vi "Sprinkler.vi"() -> ()   [LabVIEW 2020]
uses:
  SubVIs/Machine States.ctl
  Controls/Control-Indicator References.ctl
panel:
  in  "Zone Setup Array":cluster{"Zone Selector":string, "Timing":dbl}[](array[cluster])
  out "Controller Status":string
  out "Zone Indicators":T1
  in  "Water Pressure Sensor (%)":u32(slide) scale=0.0..100.0
  in  "Rain Sensor":bool
  in  "Run Selector":bool
  in  "Setup":bool
  in  "Start":bool
  in  "stop":bool
  # "Controls"
  # "Simulation Controls"
  # "Rain"
  # "No Rain"
  # "Continuous"
  # "Single"
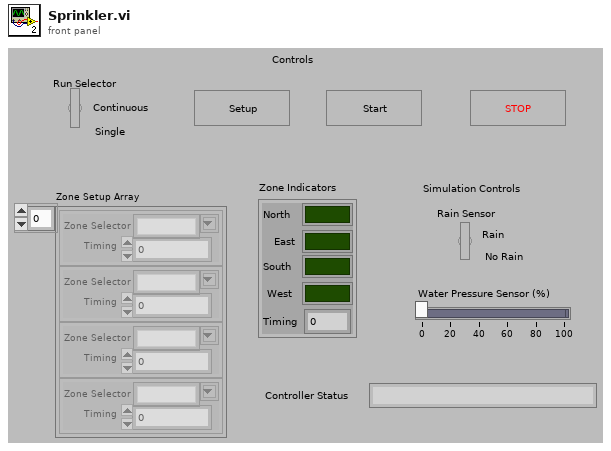
[diagram p1: front panel]
types:
  T1 = cluster{"North":bool, "East":bool, "South":bool, "West":bool, "Timing":u32}
  T2 = typedef "Control-Indicator References.ctl" = cluster{"Setup":refnum<vi>, "Start":refnum<vi>, "Controller Status":refnum<vi>, "Zone Setup Array":refnum<vi>, "Run Selector":refnum<vi>, "Rain Sensor":refnum<vi>, "Water Pressure Sensor (%)":refnum<vi>, "Zone Indicators":refnum<vi>}
  T3 = typedef "Machine States.ctl" = enum16{"Init", "Setup", "Start", "Stop", "Wait To Start", "Low Water Pressure", "Rain"}
  T4 = cluster{bool, bool, bool, bool, "Elapsed Time":dbl}
  T5 = enum8{"Enabled", "Disabled", "Disabled and Grayed Out"}
  T6 = typedef "Timer Controls.ctl" = enum16{"Reset", "Start", "Stop"}
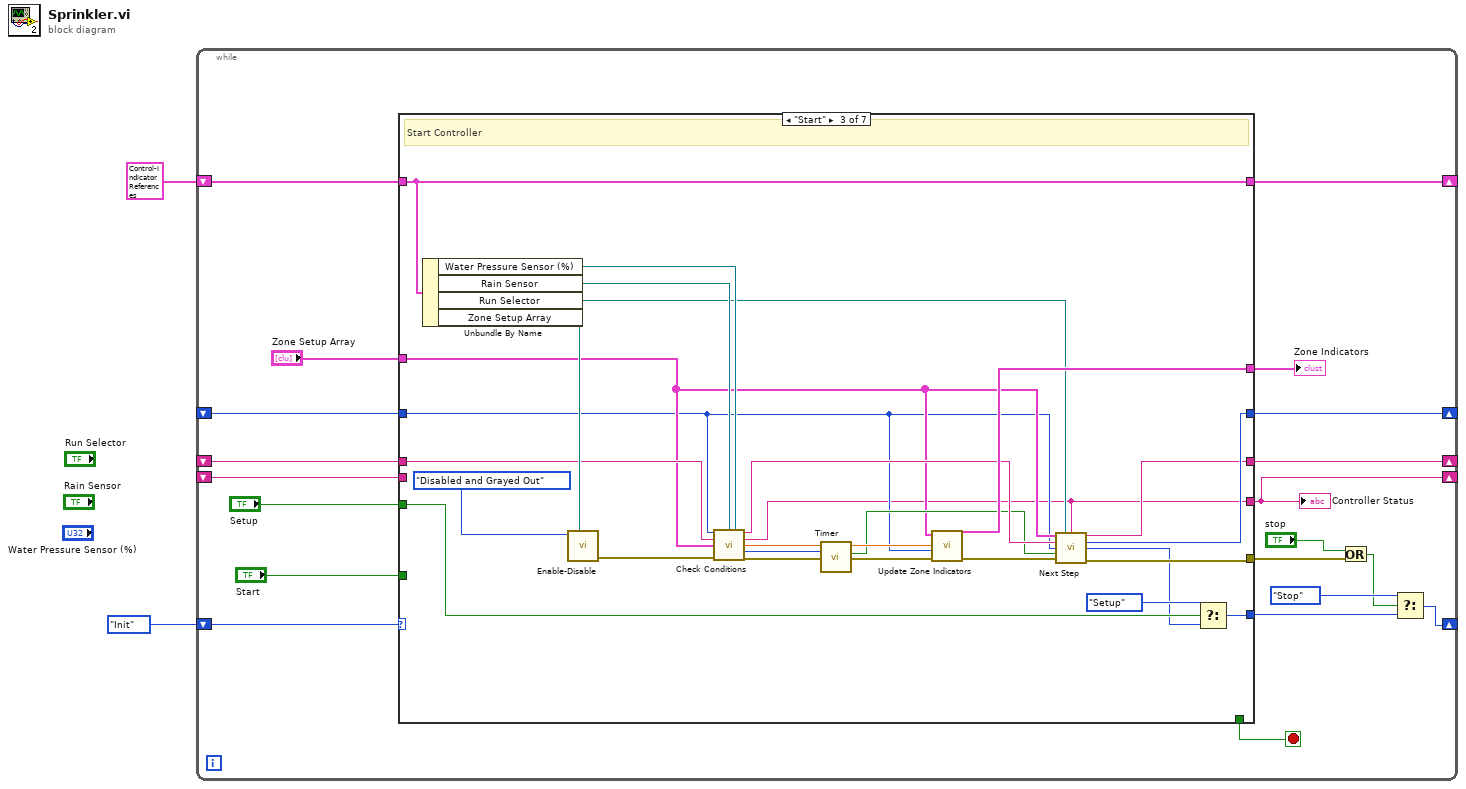
[diagram p0: block diagram]
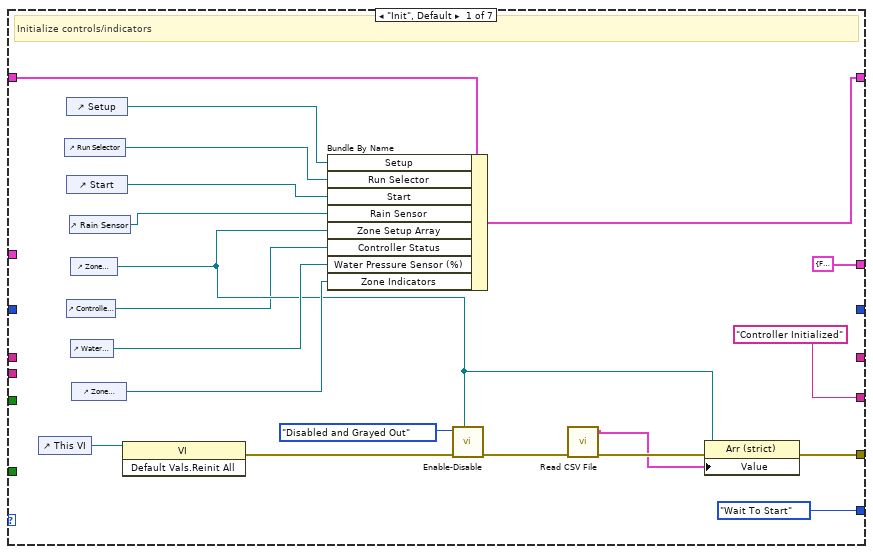
[diagram p2: hidden frame]
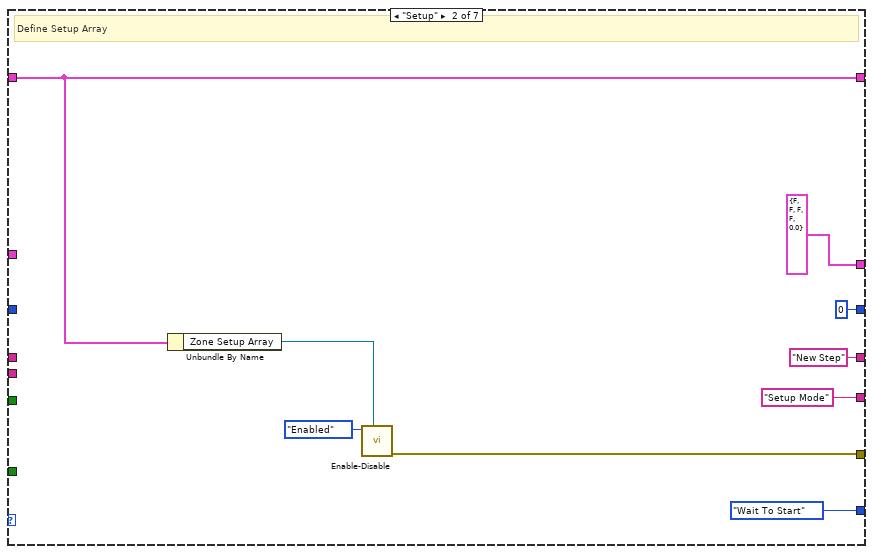
[diagram p3: hidden frame]
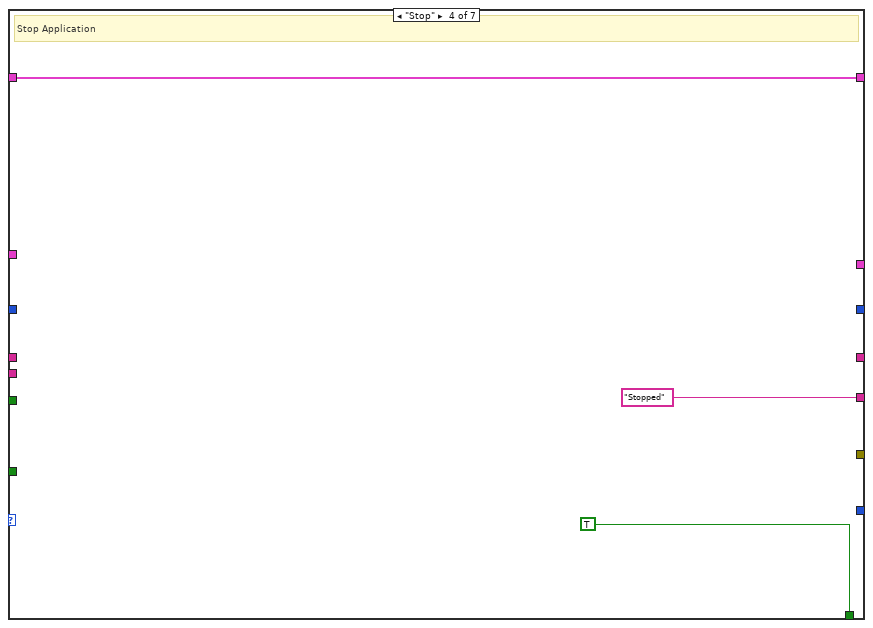
[diagram p4: hidden frame]
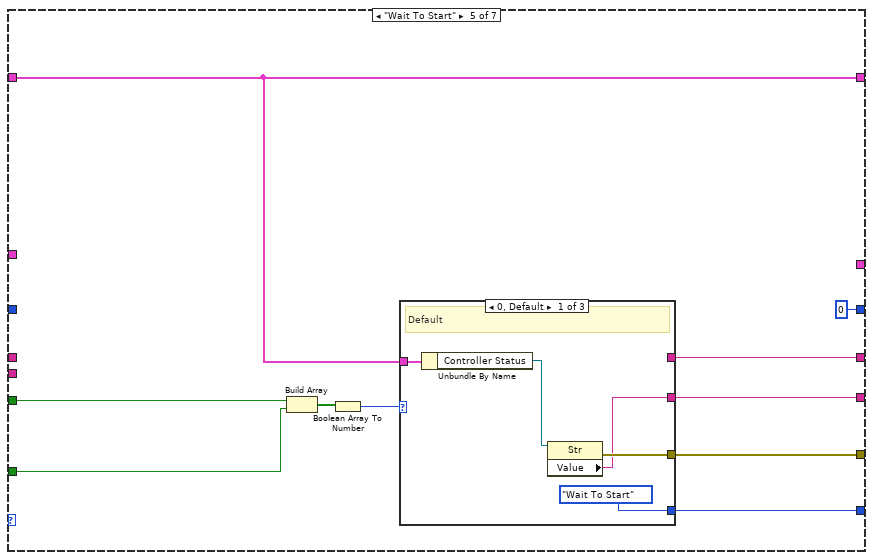
[diagram p5: hidden frame]
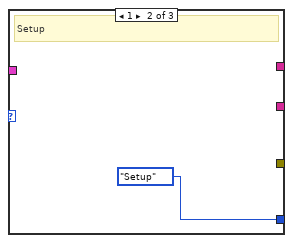
[diagram p6: hidden frame]
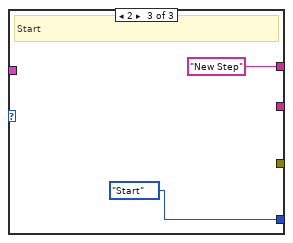
[diagram p7: hidden frame]
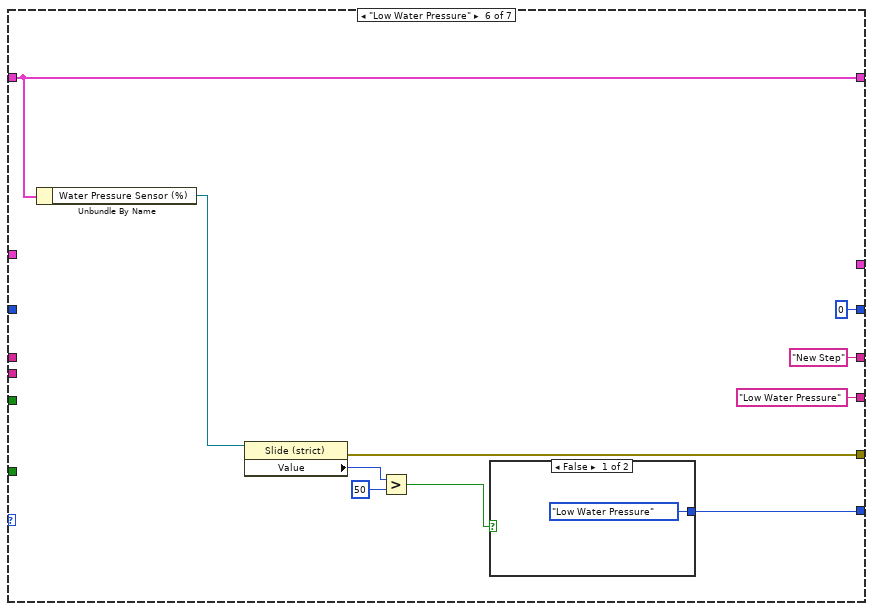
[diagram p8: hidden frame]
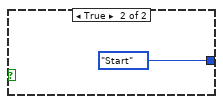
[diagram p9: hidden frame]
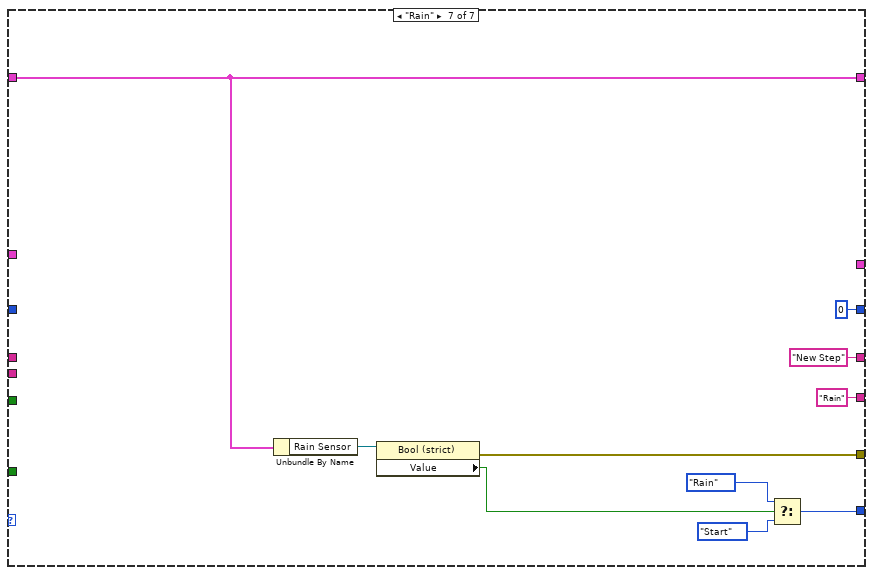
[diagram p10: hidden frame]
diagram:
  n1 = while {
    shift-right: [w18] -> _
    shift-left: Machine_States."Init" ("Enum") -> [w22]
    shift-right: [w11] -> _
    shift-left: T2 {"Setup"=refnum, "Start"=refnum, "Controller Status"=refnum, "Zone Setup Array"=refnum, "Run Selector"=refnum, "Rain Sensor"=refnum, "Water Pressure Sensor (%)"=refnum, "Zone Indicators"=refnum} -> [w21]
    shift-right: [w10] -> _
    shift-left: _ -> [w9]
    shift-right: [w7] -> _
    shift-left: _ -> [w6]
    shift-right: [w5] -> _
    shift-left: _ -> [w4]
    stop <- w17 stop-if-true
    n2 = case shown="\"Start\"" w22 {
      tunnel: w21 -> [w25 w49 w77 w78 w85 w100 w112]
      tunnel: ["Controller Initialized" ("Controller Status") "Setup Mode" ("Controller Status") w52 "Stopped" ("Controller Status") w83 "Low Water Pressure" ("Value") "Rain" ("Value")] -> w10
      tunnel: [w30 w51 w62 _ w84 w107 w116] -> w15
      tunnel: [Machine_States."Wait To Start" ("Enum") Machine_States."Wait To Start" ("f") w53 _ w86 w101 w117] -> w20
      tunnel: [_ _ _ TRUE _ _ _] -> w17
      tunnel: "Start" -> [_ _ _ _ w87 _ _]
      tunnel: "Setup" -> [_ _ w74 _ w90 _ _]
      tunnel: [w24 w49 w77 w78 w85 w100 w112] -> w11
      tunnel: w9 -> [_ _ _ _ _ _ _]
      tunnel: [_ "New Step" ("Step Status Out") w55 _ w81 "New Step" ("Step Status Out") "New Step" ("Step Status Out")] -> w7
      tunnel: "Zone Setup Array" -> [_ _ w57 _ _ _ _]
      tunnel: w6 -> [_ _ w67 _ _ _ _]
      tunnel: [_ 0 w60 _ 0 ("Step Out") 0 ("Step Out") 0 ("Step Out")] -> w5
      tunnel: w4 -> [_ _ w56 _ _ _ _]
      tunnel: [T4 {FALSE, FALSE, FALSE, FALSE, "Elapsed Time"=0.0} ("Zone Indicators") T4 {FALSE, FALSE, FALSE, FALSE, "Elapsed Time"=0.0} ("Zone Indicators") w64 _ _ _ _] -> w3
      frame "Init", Default {
        # "Initialize controls/indicators"
        n3 = control-ref of="This VI"() -> (w42:refnum<vi>)
        n4 = control-ref of="Run Selector"() -> (w40:refnum<vi>)
        n5 = control-ref of="Setup"() -> (w41:refnum<vi>)
        n6 = control-ref of="Start"() -> (w39:refnum<vi>)
        n7 = control-ref of="Controller Status"() -> (w26:refnum<vi>)
        n8 = control-ref of="Rain Sensor"() -> (w38:refnum<vi>)
        n9 = control-ref of="Zone Setup Array"() -> (w28:refnum<vi>)
        n10 = control-ref of="Water Pressure Sensor (%)"() -> (w37:refnum<vi>)
        n11 = control-ref of="Zone Indicators"() -> (w29:refnum<vi>)
        n12 = invoke class="VI" method="Default Vals.Reinit All"(reference=w42) -> (error out=w36:errorcluster)  [unwired: 2 in, 2 out]
        n13 = Bundle By Name(cluster=w25, "Setup"=w41, "Run Selector"=w40, "Start"=w39, "Rain Sensor"=w38, "Zone Setup Array"=w28, "Controller Status"=w26, "Water Pressure Sensor (%)"=w37, "Zone Indicators"=w29) -> (w24:T2)
        n14 = call "Enable-Disable.vi"("Reference in"=w28, "error in (no error)"=w36, "E/D"=T5."Disabled and Grayed Out") -> ("error out"=w32:errorcluster)  [unwired: 8 in]
        n15 = call "Read CSV File.vi"("error in"=w32) -> ("error out"=w31:errorcluster, "Zone Setup Array"=w27:cluster{"Zone Selector":string, "Timing":dbl}[])  [unwired: 9 in]
        n16 = property class="Arr (strict)"(reference=w28, error in=w31, "Value"=w27) -> (error out=w30:errorcluster)  [unwired: 1 out]
      }
      frame "Setup" {
        # "Define Setup Array"
        n17 = Unbundle By Name(w49) -> ("Zone Setup Array"=w44:refnum<vi>)
        n18 = call "Enable-Disable.vi"("Reference in"=w44, "E/D"=T5."Enabled") -> ("error out"=w51:errorcluster)  [unwired: 9 in]
      }
      frame "Start" {
        # "Start Controller"
        n19 = Unbundle By Name(w77) -> ("Water Pressure Sensor (%)"=w71:refnum<vi>, "Rain Sensor"=w72:refnum<vi>, "Run Selector"=w58:refnum<vi>, "Zone Setup Array"=w73:refnum<vi>)
        n20 = call "Enable-Disable.vi"("Reference in"=w73, "E/D"=T5."Disabled and Grayed Out") -> ("error out"=w70:errorcluster)  [unwired: 9 in]
        n21 = call "Check Conditions.vi"("Zone"=w56, "Rain Sensor"=w72, "Water Pressure Sensor (%)"=w71, "Step Status In"=w67, "Zone Setup Array in"=w57, "error in"=w70) -> ("Step Status Out"=w61:string, "Controller Status"=w52:string, "Zone Timer"=w69:dbl, "Timer Status"=w68:T6, "error out"=w65:errorcluster)  [unwired: 5 in]
        n22 = call "Timer.vi"("Timer Control"=w68, "Time Target"=w69) -> ("Time completed?"=w59:bool, "Elapsed Time"=w66:dbl)  [unwired: 8 in]
        n23 = call "Update Zone Indicators.vi"("error in"=w65, "Step"=w56, "Elapsed Time"=w66, "Zone Setup Array"=w57) -> ("error out"=w63:errorcluster, "Zone Indicators"=w64:T4)  [unwired: 6 in]
        n24 = call "Next Step.vi"("Zone Setup Array in"=w57, "Run Selector Reference"=w58, "Controller Status"=w52, "Step Status In"=w61, "Step In"=w56, "Time completed?"=w59, "error in"=w63) -> ("Step Status Out"=w55:string, "Step Out"=w60:i32, "Machine State"=w54:T3, "error out"=w62:errorcluster)  [unwired: 5 in]
        n25 = Select(t=Machine_States."Setup", s=w74, f=w54) -> (s? t:f=w53:T3)
      }
      frame "Stop" {
        # "Stop Application"
      }
      frame "Wait To Start" {
        n26 = Build Array(w90, w87) -> (w89:bool[])
        n27 = Boolean Array To Number(Boolean array=w89) -> (number=w88:u32)
        n28 = case shown="0, Default" w88 {
          tunnel: [Machine_States."Wait To Start" ("f") Machine_States."Setup" ("f") Machine_States."Start" ("f")] -> w86
          tunnel: w85 -> [w93 _ _]
          tunnel: [w92 _ _] -> w84
          tunnel: [w91 _ _] -> w83
          tunnel: [_ _ "New Step" ("Step Status Out")] -> w81
          frame 0, Default {
            # "Default"
            n29 = Unbundle By Name(w93) -> ("Controller Status"=w94:refnum<vi>)
            n30 = property class="Str"(reference=w94) -> (error out=w92:errorcluster, "Value"=w91:string)  [unwired: 1 in, 1 out]
          }
          frame 1 {
            # "Setup"
          }
          frame 2 {
            # "Start"
          }
        }
      }
      frame "Low Water Pressure" {
        n31 = Unbundle By Name(w100) -> ("Water Pressure Sensor (%)"=w108:refnum<vi>)
        n32 = property class="Slide (strict)"(reference=w108) -> (error out=w107:errorcluster, "Value"=w106:u32)  [unwired: 1 in, 1 out]
        n33 = Greater?(x=w106, y=u32 50) -> (0:w104:bool)
        n34 = case shown="False" w104 {
          tunnel: [Machine_States."Low Water Pressure" ("f") Machine_States."Start" ("f")] -> w101
          frame False {
          }
          frame True {
          }
        }
      }
      frame "Rain" {
        n35 = Unbundle By Name(w112) -> ("Rain Sensor"=w118:refnum<vi>)
        n36 = property class="Bool (strict)"(reference=w118) -> (error out=w116:errorcluster, "Value"=w115:bool)  [unwired: 1 in, 1 out]
        n37 = Select(t=Machine_States."Rain", s=w115, f=Machine_States."Start" ("t")) -> (s? t:f=w117:T3)
      }
    }
    "Zone Indicators" <- w3
    "Controller Status" <- w10
    n38 = Or(x="stop", y=w15) -> (x .or. y?=w14:bool)
    n39 = Select(t=Machine_States."Stop", s=w14, f=w20) -> (s? t:f=w18:T3)
  }
